vi "tree excel.vi"   [LabVIEW 2013]
doc: "Philips Research, COS/TMA aug 2000"
panel:
  # "EXCEL TOOLKIT v1.1\n\nSEE DIAGRAM FOR TREE OVERVIEW..."
types:
  T1 = enum16{"open workbook as template", "open workbook from file", "create new workbook"}
  T2 = typedef "excel Object Reference.ctl" = refnum<k1>
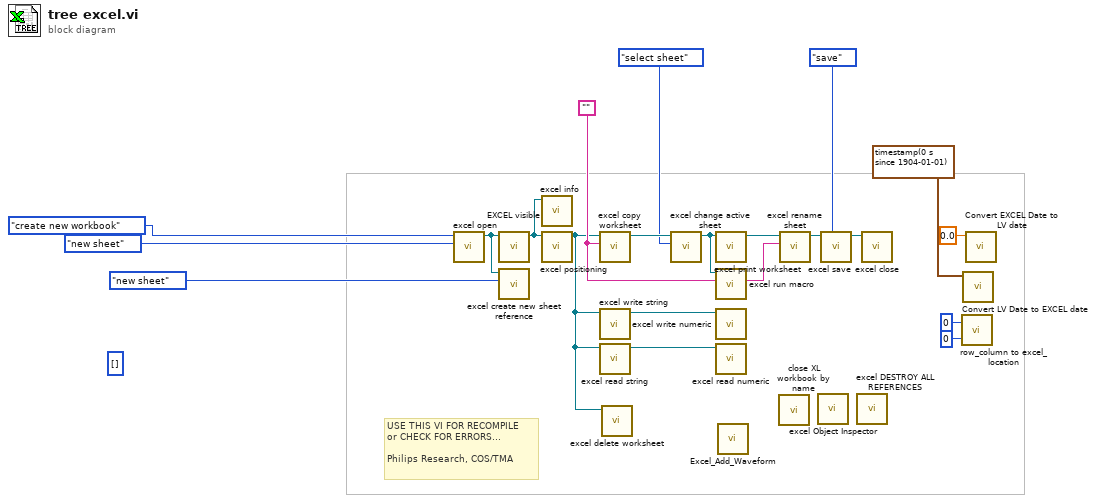
[diagram p0: block diagram]
diagram:
  w6 = ""
  (unwired) i32[] [] ("array size(s)\n  - #rows\n  - #columns")
  # "USE THIS VI FOR RECOMPILE\nor CHECK FOR ERRORS...\n\nPhilips Research, COS/TMA"
  n1 = call "excel open.vi"("mode_sheet"=enum16{"new sheet", "select sheet"}."new sheet", "mode_workbook"=T1."create new workbook") -> ("reference"=w16:T2)  [unwired: 8 in, 1 out]
  n2 = call "EXCEL visible.vi"("reference"=w16) -> ("duplicate reference"=w15:T2)  [unwired: 9 in, 1 out]
  n3 = call "excel create new sheet reference.vi"("mode_sheet"=enum16{"new sheet", "select sheet"}."new sheet", "reference"=w16) -> ()  [unwired: 7 in, 3 out]
  n4 = call "excel info.vi"("reference"=w15) -> ()  [unwired: 7 in, 4 out]
  n5 = call "excel positioning.vi"("reference"=w15) -> ("duplicate reference"=w5:T2)  [unwired: 9 in, 1 out]
  n6 = call "excel copy worksheet.vi"("dest. sheetname"=w6, "reference"=w5) -> ("reference out"=w20:T2)  [unwired: 8 in, 1 out]
  n7 = call "excel write string.vi"("reference"=w5) -> ("duplicate reference"=w14:T2)  [unwired: 9 in, 1 out]
  n8 = call "excel read string.vi"("reference"=w5) -> ("duplicate reference"=w13:T2)  [unwired: 7 in, 3 out]
  n9 = call "excel delete worksheet.vi"("reference"=w5) -> ()  [unwired: 9 in, 2 out]
  n10 = call "excel change active sheet.vi"("mode_sheet"=enum16{"new sheet", "select sheet"}."select sheet", "reference"=w20) -> ("duplicate reference"=w12:T2)  [unwired: 8 in, 1 out]
  n11 = call "excel print worksheet.vi"("reference"=w12) -> ("duplicate reference"=w19:T2)  [unwired: 9 in, 1 out]
  n12 = call "excel run macro.vi"("macro name"=w6, "reference"=w12) -> ()  [unwired: 8 in, 2 out]
  n13 = call "excel write numeric.vi"("reference"=w14) -> ()  [unwired: 9 in, 2 out]
  n14 = call "excel read numeric.vi"("reference"=w13) -> ()  [unwired: 7 in, 4 out]
  n15 = call "Excel_Add_Waveform.vi"() -> ()  [unwired: 10 in, 2 out]
  n16 = call "close XL workbook by name.vi"() -> ()  [unwired: 11 in, 1 out]
  n17 = call "excel rename sheet.vi"("new name"=w6, "reference"=w19) -> ("duplicate reference"=w18:T2)  [unwired: 6 in, 3 out]
  n18 = call "excel Object Inspector.vi"() -> ()  [unwired: 1 in]
  n19 = call "excel save.vi"("mode_save"=enum16{"save", "save as", "save a copy as"}."save", "reference"=w18) -> ("duplicate reference"=w17:T2)  [unwired: 8 in, 1 out]
  n20 = call "excel DESTROY ALL REFERENCES.vi"() -> ()  [unwired: 1 in]
  n21 = call "excel close.vi"("reference"=w17) -> ()  [unwired: 6 in, 1 out]
  n22 = call "row_column to excel_location.vi"("Column"=0, "Row"=0) -> ()  [unwired: 1 out]
  n23 = call "Convert LV Date to EXCEL date.vi"("LV time stamp"=timestamp(0 s since 1904-01-01)) -> ()  [unwired: 9 in, 2 out]
  n24 = call "Convert EXCEL Date to LV date.vi"("Excel Timestamp"=0.0) -> ()  [unwired: 9 in, 2 out]
